vi "Contains Entry.vi"(8 "error in":errorcluster, 10 "ID":string, 11 "Object Dictionary in":refnum<class "Object Dictionary.lvclass">) -> (0 "error out":errorcluster, 1 "Index":i32, 2 "Found?":bool, 3 "Object Dictionary out":refnum<class "Object Dictionary.lvclass">)   [LabVIEW 2024, in "EDS.lvlib" / "Object Dictionary.lvclass"]
uses:
  Object Dictionary.lvclass
  Object Dictionary.lvclass/Object Dictionary.ctl
  Object Entry/Object Entry.lvclass/Object Entry.ctl
  Object Entry/Get ID.vi
  Object Entry/Object Entry.lvclass
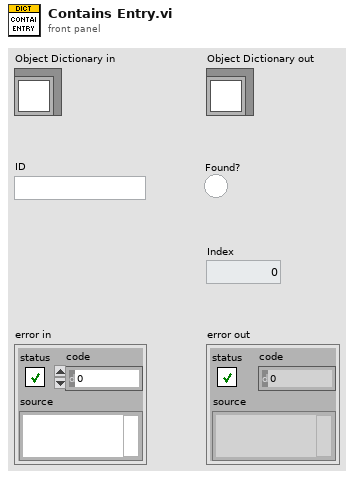
[diagram p1: front panel]
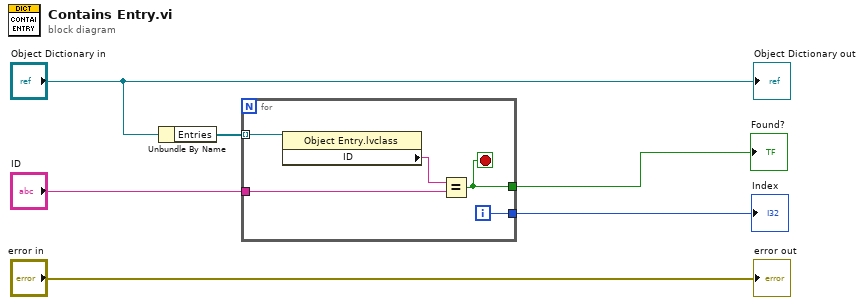
[diagram p0: block diagram]
diagram:
  n1 = Unbundle By Name("Object Dictionary in") -> ("Entries"=w4:refnum<class "Object Entry.lvclass">[])
  n2 = for {
    tunnel: w4 -> [w10] mode=indexing
    tunnel: "ID" -> [w11]
    tunnel: [w8] -> w1
    tunnel: [w7] -> w2
    i -> [w8]
    stop <- w7 stop-if-true
    n3 = property class="Object Entry.lvclass"(reference=w10) -> ("ID"=w9:string)  [unwired: 1 in, 2 out]
    n4 = Equal?(x=w9, y=w11) -> (x = y?=w7:bool)
  }
  "Found?" <- w2
  "Index" <- w1
  "error out" <- "error in"
  "Object Dictionary out" <- "Object Dictionary in"
